vi "3차보간.vi"() -> ()   [LabVIEW 2016]
uses:
  <vilib>/imath/engines/lvmath2/RunTimeEngine/IndexRead/NIMS M(S).vi
  <instcachedir>/0/NIMS M(S)_B826C018497E4940AE96BD27B540B6FB.lvgen/NIMS M(S)_B826C018497E4940AE96BD27B540B6FB_000.vi
  <vilib>/imathl/engines/lvmath/Functions/Error Handling/Create Error.vi
  <vilib>/imath/engines/lvmath2/RunTimeEngine/BuiltInFunctions/deg_to_rad/NIMS_deg_to_rad.vi
  <instcachedir>/0/NIMS_deg_to_rad_4A81D684CE8D4DD79924F5AB74D756E1.lvgen/NIMS_deg_to_rad_4A81D684CE8D4DD79924F5AB74D756E1_001.vi
  <vilib>/imath/engines/lvmath2/RunTimeEngine/IndexRead/NIMS M($,S).vi
  <instcachedir>/0/NIMS M($,S)_3E5749BBB62E49528D4765A77F1F6D98.lvgen/NIMS M($,S)_3E5749BBB62E49528D4765A77F1F6D98_000.vi
  <instcachedir>/0/NIMS_deg_to_rad_4A81D684CE8D4DD79924F5AB74D756E1.lvgen/NIMS_deg_to_rad_4A81D684CE8D4DD79924F5AB74D756E1_002.vi
  <vilib>/imath/engines/lvmath2/RunTimeEngine/ArithmeticOperatorToken/NIMS_ArithmeticOperator_times.vi
  <instcachedir>/0/NIMS_ArithmeticOperator_times_953B34F74CAC448FB707D816A29CC5F0.lvgen/NIMS_ArithmeticOperator_times_953B34F74CAC448FB707D816A29CC5F0_000.vi
  <vilib>/imath/engines/lvmath2/RunTimeEngine/RowToken/NIMS_RowToken_CV_CV.vi
  <instcachedir>/0/NIMS_RowToken_CV_CV_5546A0B1CA2C4E49826F811B9C073FB0.lvgen/NIMS_RowToken_CV_CV_5546A0B1CA2C4E49826F811B9C073FB0_000.vi
  <vilib>/imath/engines/lvmath2/RunTimeEngine/IndexRead/NIMS V(S).vi
  <instcachedir>/0/NIMS V(S)_0488751826AF41519A22953C041130DC.lvgen/NIMS V(S)_0488751826AF41519A22953C041130DC_000.vi
  <vilib>/imath/engines/lvmath2/RunTimeEngine/ErrorHandling/NIMS_Create Error From Enums.vi
  <vilib>/imath/engines/lvmath2/RunTimeEngine/RowToken/NIMS_RowToken_M_CV.vi
  <instcachedir>/0/NIMS_RowToken_M_CV_FA79F1D1D17D44459F3ED8E09EE8B625.lvgen/NIMS_RowToken_M_CV_FA79F1D1D17D44459F3ED8E09EE8B625_000.vi
  <vilib>/imath/engines/lvmath2/RunTimeEngine/ArithmeticOperatorToken/NIMS_ArithmeticOperator_leftdivmx-internal.vi
  <instcachedir>/0/NIMS_ArithmeticOperator_leftdivmx-internal_7B09604CE770471B80B1C10AF4734F6D.lvgen/NIMS_ArithmeticOperator_leftdivmx-internal_7B09604CE770471B80B1C10AF4734F6D_000.vi
  <vilib>/imath/engines/lvmath2/RunTimeSupport/NIMS_Get Column Vector - Matrix.vi
  <instcachedir>/0/NIMS_Get Column Vector - Matrix_9A41694D383F4F97A368BCDCEE24DC60.lvgen/NIMS_Get Column Vector - Matrix_9A41694D383F4F97A368BCDCEE24DC60_000.vi
  <vilib>/imath/engines/lvmath2/RunTimeSupport/NIMS_Complex To Real.vi
  <instcachedir>/0/NIMS_Complex To Real_A9DD49CC305F495FA24B9F5762C73A31.lvgen/NIMS_Complex To Real_A9DD49CC305F495FA24B9F5762C73A31_001.vi
  <vilib>/imath/engines/lvmath2/RunTimeEngine/BuiltInFunctions/rad_to_deg/NIMS_rad_to_deg.vi
  <instcachedir>/0/NIMS_rad_to_deg_A39AFCDDC8C049FCADAAB7FC30B9F5AA.lvgen/NIMS_rad_to_deg_A39AFCDDC8C049FCADAAB7FC30B9F5AA_001.vi
  <vilib>/imath/engines/lvmath2/RunTimeEngine/NodeEndStatement/NIMS_NodeEndStatement_Output.vi
  <instcachedir>/0/NIMS_NodeEndStatement_Output_53EC0D466D134D7ABD903AC30B43404B.lvgen/NIMS_NodeEndStatement_Output_53EC0D466D134D7ABD903AC30B43404B_001.vi
  <instcachedir>/0/NIMS_NodeEndStatement_Output_53EC0D466D134D7ABD903AC30B43404B.lvgen/NIMS_NodeEndStatement_Output_53EC0D466D134D7ABD903AC30B43404B_005.vi
  <instcachedir>/0/NIMS_NodeEndStatement_Output_53EC0D466D134D7ABD903AC30B43404B.lvgen/NIMS_NodeEndStatement_Output_53EC0D466D134D7ABD903AC30B43404B_002.vi
  <vilib>/imath/engines/lvmath2/RunTimeEngine/ErrorHandling/NIMS_Finalize Error.vi
panel:
  out "SA":cdb
  out "D":dbl[](array[numeric])
  out "C":dbl[](array[numeric])
  out "B":dbl[][](array[numeric])
  out "A":dbl[](array[numeric])
  out "LC_Nav":dbl[][](array[numeric])
  in  "GPS":dbl[][](array[numeric])
  in  "Lane Center":dbl[][](array[numeric])
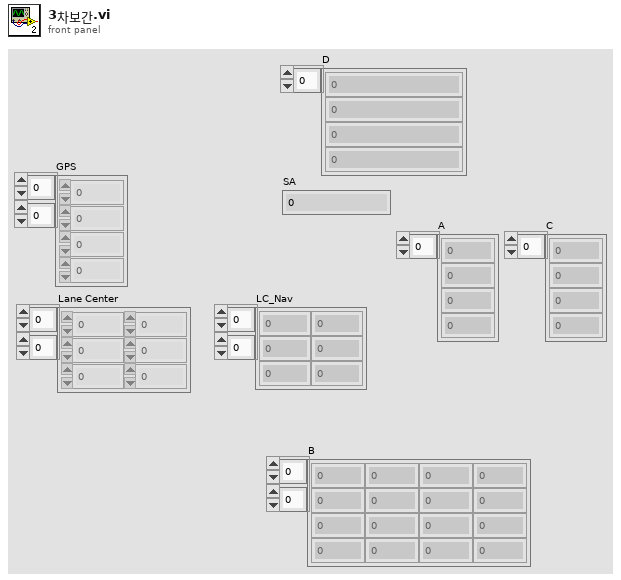
[diagram p1: front panel]
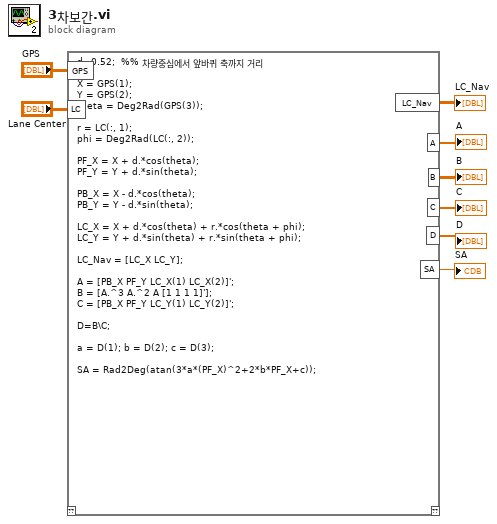
[diagram p0: block diagram]
diagram:
  n1 = mathscript code="d=0.52;  %% 차량중심에서 앞바퀴 축까지 거리\n\nX = GPS(1);\nY = GPS(2);\ntheta = Deg2Rad(GPS(3));\n\nr = LC(:, 1);\nphi = Deg2Rad(LC(:, 2));\n\nPF_X = X + d.*cos(theta);\nPF_Y = Y + d.*sin(theta);\n\nPB_X = X - d.*cos(theta);\nPB_Y = Y - d.*sin(theta);\n\nLC_X = X + d.*cos(theta) + r.*cos(theta + phi);\nLC_Y = Y + d.*sin(theta) + r.*sin(theta + phi);\n\nLC_Nav = [LC_X LC_Y];\n\nA = [PB_X PF_Y LC_X(1) LC_X(2)]';\nB = [A.^3 A.^2 A [1 1 1 1]'];\nC = [PB_X PF_Y LC_Y(1) LC_Y(2)]';\n\nD=B\\C;\n\na = D(1); b = D(2); c = D(3);\n\nSA = Rad2Deg(atan(3*a*(PF_X)^2+2*b*PF_X+c));"("GPS"="GPS", "LC"="Lane Center") -> ("LC_Nav"=→"LC_Nav":dbl[][], "A"=→"A":dbl[], "B"=→"B":dbl[][], "C"=→"C":dbl[], "D"=→"D":dbl[], "SA"=→"SA":dbl)  [unwired: 1 in, 1 out]
